vi "Set Channel Properties.vi"(8 "error in (no error)":errorcluster, 10 "Group":refnum<class "Group DBL.lvclass">, 11 "File in":refnum<k34>) -> (0 "error out":errorcluster, 1 "Channel Names":string[](array[string]), 2 "Group Name":string, 3 "File":refnum<k34>)   [LabVIEW 2020, in "VolatusData.lvlib" / "Data Logger DBL Module.lvclass"]
uses:
  Data Logger DBL Module.lvclass
  lv-vecto/Vecto/Group/Group.lvclass
  lv-vecto/Vecto/Group Config/Group Config.lvclass
  lv-vecto/Vecto/Channel Config/Channel Config.lvclass
  lv-vecto/Vecto/Group DBL/Group DBL.lvclass
  C:/dev/lv20CE/relink/lv-vecto/Vecto/Group/Group.lvclass
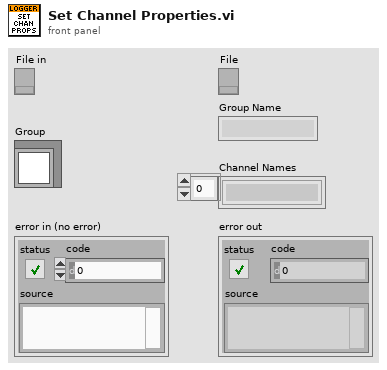
[diagram p1: front panel]
types:
  T1 = typedef "VectoConfig.lvlib/Publish Config.ctl" = cluster{"Address":string, "Port":u16}
  T2 = typedef "VectoConfig.lvlib/Channel Info.ctl" = cluster{"Name":string, "Group":string, "Owning Node":string, "Owning Task":string, "Resource":string}
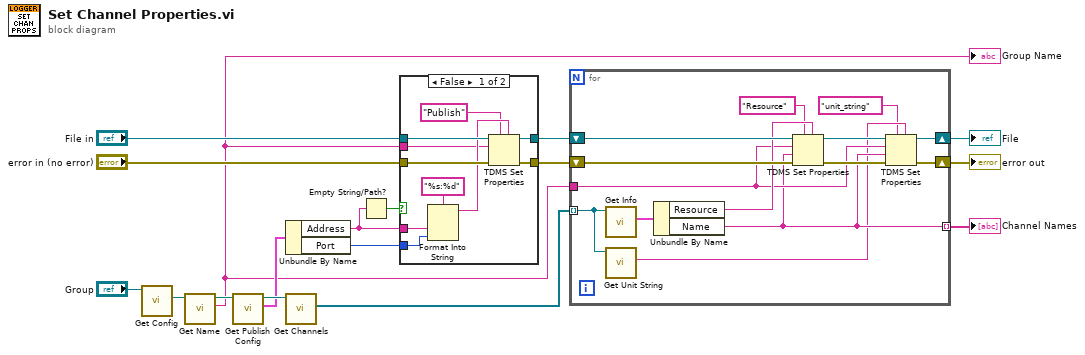
[diagram p0: block diagram]
diagram:
  n1 = call "Get Config.vi"("Group in"="Group") -> ("Config"=w15:refnum<class "Group Config.lvclass">)  [unwired: 8 in, 2 out]
  n2 = call "Get Name.vi"("Group Config in"=w15) -> ("Name"=w4:string, "Group Config out"=w14:refnum<class "Group Config.lvclass">)  [unwired: 8 in, 1 out]
  "Group Name" <- w4
  n3 = call "Get Publish Config.vi"("Group Config in"=w14) -> ("Publish Config"=w13:T1, "Group Config out"=w17:refnum<class "Group Config.lvclass">)  [unwired: 8 in, 1 out]
  n4 = Unbundle By Name(w13) -> ("Address"=w11:string, "Port"=w10:u16)
  n5 = call "Get Channels.vi"("Group Config in"=w17) -> ("Channels"=w5:refnum<class "Channel Config.lvclass">[])  [unwired: 8 in, 2 out]
  n6 = Empty String/Path?(string/path=w11) -> (empty?=w12:bool)
  n7 = case shown="False" w12 {
    tunnel: w11 -> [w27 _]
    tunnel: w10 -> [w26 _]
    tunnel: "File in" -> [w24 w29]
    tunnel: "error in (no error)" -> [w23 w28]
    tunnel: w4 -> [w20 _]
    tunnel: [w19 w28] -> w6
    tunnel: [w18 w29] -> w7
    frame False {
      n8 = Format Into String(format string="%s:%d", w27, w26) -> (resulting string=w22:string)  [unwired: 2 in, 1 out]
      n9 = TDMS Set Properties(5:w22, 7:"Publish" ("property names"), 8:w23, 10:w20, 11:w24) -> (0:w19:errorcluster, 3:w18:refnum<k34>)  [unwired: 1 in, 2 out]
    }
    frame True {
    }
  }
  n10 = for {
    shift-right: [w31] -> w2
    shift-left: w7 -> [w43]
    shift-right: [w30] -> w3
    shift-left: w6 -> [w42]
    tunnel: w5 -> [w38] mode=indexing
    tunnel: w4 -> [w35]
    tunnel: [w34] -> w1 mode=indexing
    n11 = call "Get Info.vi"("Channel Config in"=w38) -> ("Info"=w41:T2)  [unwired: 8 in, 2 out]
    n12 = call "Get Unit String.vi"("Channel Config in"=w38) -> ("Unit String"=w33:string)  [unwired: 8 in, 2 out]
    n13 = Unbundle By Name(w41) -> ("Resource"=w40:string, "Name"=w34:string)
    n14 = TDMS Set Properties(5:w40, 7:"Resource" ("property names"), 8:w42, 9:w34, 10:w35, 11:w43) -> (0:w37:errorcluster, 3:w36:refnum<k34>)  [unwired: 2 out]
    n15 = TDMS Set Properties(5:w33, 7:"unit_string" ("property names"), 8:w37, 9:w34, 10:w35, 11:w36) -> (0:w30:errorcluster, 3:w31:refnum<k34>)  [unwired: 2 out]
  }
  "error out" <- w3
  "File" <- w2
  "Channel Names" <- w1
